vi "Read Key.vi"(6 "Key Name":string, 8 "error in":errorcluster, 11 "Config in":refnum<class "Config.lvclass">) -> (0 "error out":errorcluster, 2 "Key Value":string, 3 "Config out":refnum<class "Config.lvclass">)   [LabVIEW 2023, in "Config.lvlib" / "Config.lvclass"]
uses:
  Config.lvclass
  Config.lvclass/Config.ctl
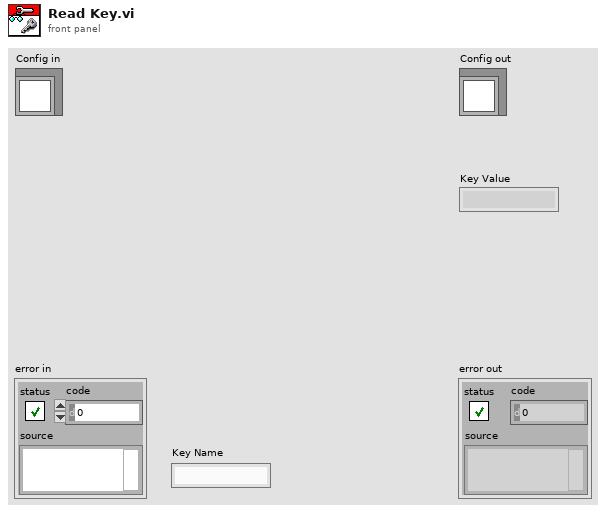
[diagram p1: front panel]
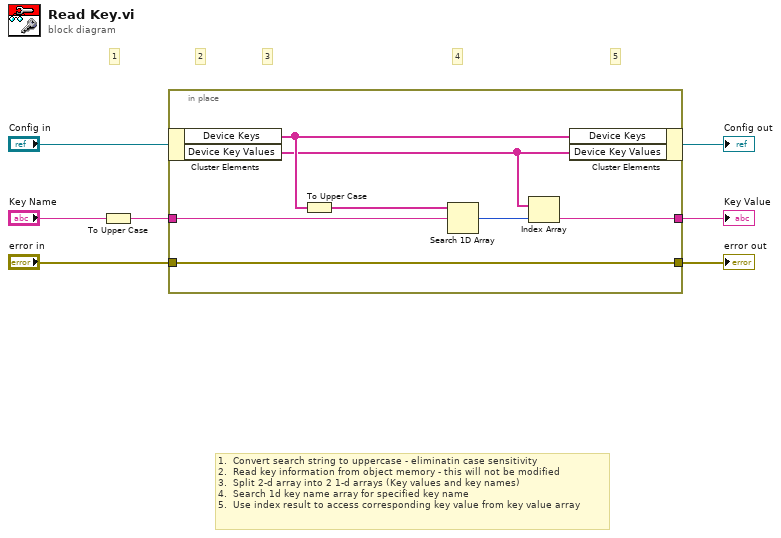
[diagram p0: block diagram]
diagram:
  # "1.  Convert search string to uppercase - eliminatin case sensitivity\n2.  Read key information from object memory - this will not be modified\n3.  Split 2-d array into 2 1-d arrays (Key values and key names)\n4.  Search 1d key name array for specified key name\n5.  Use index result to access corresponding key value from key value array"
  # "5"
  # "4"
  # "3"
  # "2"
  # "1"
  n1 = To Upper Case(1:"Key Name") -> (0:w1:string)
  n2 = in-place {
    in-place-border: w1 -> [w14]
    in-place-border: "error in" -> [w13]
    in-place-border: [w13] -> w3
    in-place-border: [w9] -> w2
    n3 = in-place-cluster #1("Config in") -> ("Device Keys"=w12:string[], "Device Key Values"=w10:string[])
    n4 = To Upper Case(1:w12) -> (0:w8:string[])
    n5 = Search 1D Array(1D array=w8, element=w14) -> (index of element=w11:i32)  [unwired: 1 in]
    n6 = Index Array(array=w10, index=w11) -> (element=w9:string)
    n7 = in-place-cluster #1("Device Keys"=w12, "Device Key Values"=w10) -> (→"Config out":refnum<class "Config.lvclass">)
  }
  "error out" <- w3
  "Key Value" <- w2
